vi "Queue - Create.vi"(8 "error in":errorcluster, 11 "Queue Name":string) -> (0 "error out":errorcluster)   [LabVIEW 2024, in "QMH Messaging.lvlib"]
uses:
  QMH Messaging.lvlib
  General Type Defs/FGV States.ctl
  General Type Defs/General Type Defs.lvlib
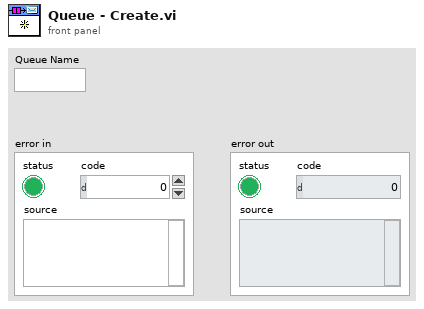
[diagram p1: front panel]
types:
  T1 = typedef "General Type Defs.lvlib/FGV States.ctl" = enum16{"Create", "Get", "Destroy"}
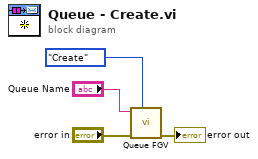
[diagram p0: block diagram]
diagram:
  n1 = call "Queue FGV.vi"("FGV States"=FGV_States."Create", "error in"="error in", "Queue Name"="Queue Name") -> ("error out"=→"error out":errorcluster)  [unwired: 7 in, 1 out]
